vi "Display Error.vi"(8 "error in (no error)":errorcluster, 11 "Application Manager":refnum<k7>) -> (0 "error out":errorcluster)   [LabVIEW 2010, in "TS Simple LabVIEW OI Dependencies.lvlib"]
uses:
  TS Simple LabVIEW OI Dependencies.lvlib
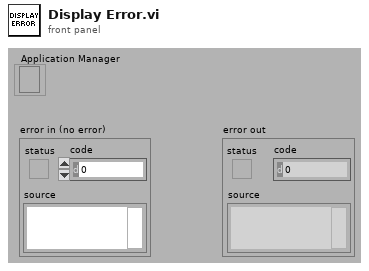
[diagram p1: front panel]
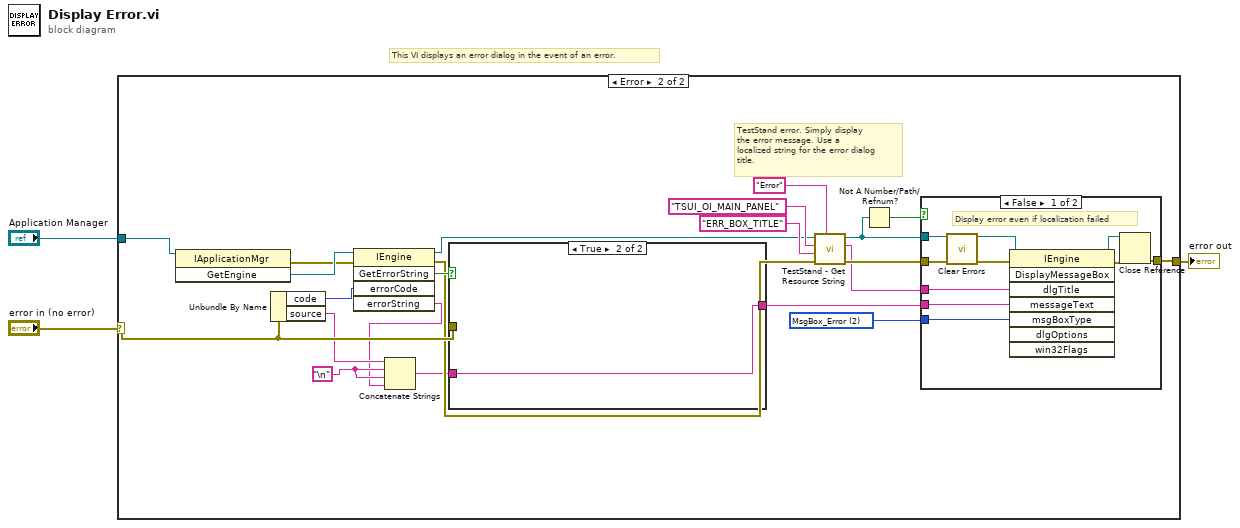
[diagram p0: block diagram]
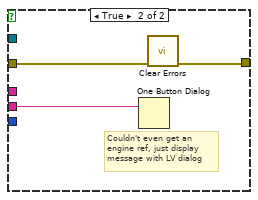
[diagram p3: hidden frame]
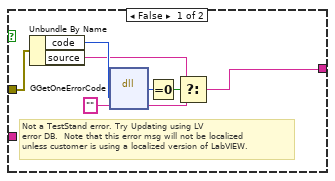
[diagram p4: hidden frame]
diagram:
  # "This VI displays an error dialog in the event of an error."
  n1 = case shown="Error" "error in (no error)" {
    selector: "error in (no error)" -> [w4 w24]
    tunnel: [w4 w16] -> w2
    tunnel: "Application Manager" -> [_ w17]
    frame No Error {
    }
    frame Error {
      w6 = "\n"
      w12 = 2 items=["MsgBox_Warning", "MsgBox_Information", "MsgBox_Error", "MsgBox_Custom"] ("msgBoxType")
      # "TestStand error. Simply display\nthe error message. Use a\nlocalized string for the error dialog\ntitle."
      n2 = invoke class="IApplicationMgr" method="GetEngine"(reference=w17) -> (error out=w22:errorcluster, "GetEngine"=w23:refnum<k7>)  [unwired: 2 in, 1 out]
      n3 = Unbundle By Name(w24) -> ("code"=w26:i32, "source"=w7:string)
      n4 = invoke class="IEngine" method="GetErrorString"(reference=w23, error in=w22, "errorCode"=w26) -> (reference out=w18:refnum<k7>, error out=w19:errorcluster, "GetErrorString"=w25:bool, "errorString"=w5:string)  [unwired: 2 in, 1 out]
      n5 = Concatenate Strings(w7, w6, w6, w5) -> (w8:string)
      n6 = case shown="True" w25 {
        tunnel: w24 -> [w40 _]
        tunnel: [w39 w47] -> w13
        tunnel: w8 -> [_ w47]
        frame False {
          # "Not a TestStand error. Try Updating using LV\nerror DB.  Note that this error msg will not be localized\nunless customer is using a localized version of LabVIEW."
          n7 = Unbundle By Name(w40) -> ("code"=w42:i32, "source"=w41:string)
          n8 = dll-call lib="LabVIEW" fn="GGetOneErrorCode"("errorCode"=w42, "" ("input param")) -> (w45:u8, w43:string)  [unwired: 4 in, 2 out]
          n9 = Equal To 0?(x=w45) -> (x = 0?=w44:bool)
          n10 = Select(t=w41, s=w44, f=w43) -> (s? t:f=w39:string)
        }
        frame True {
        }
      }
      n11 = call <vilib>:"TestStand - Get Resource String.vi"("Default String"="Error", "error in (no error)"=w19, "Symbol"="ERR_BOX_TITLE", "Category"="TSUI_OI_MAIN_PANEL", "Engine Reference In"=w18) -> ("error out"=w15:errorcluster, "Resource String"=w14:string, "Engine Reference Out"=w11:refnum<k7>)  [unwired: 4 out]
      n12 = Not A Number/Path/Refnum?(number/path/refnum=w11) -> (NaN/Path/Refnum?=w10:bool)
      n13 = case shown="False" w10 {
        tunnel: [w35 w36] -> w16
        tunnel: w12 -> [w34 _]
        tunnel: w14 -> [w33 _]
        tunnel: w11 -> [w32 _]
        tunnel: w15 -> [w28 w37]
        tunnel: w13 -> [w29 w38]
        frame False {
          # "Display error even if localization failed"
          n14 = call <vilib>:"Clear Errors.vi"("error in (no error)"=w28) -> ("error out"=w27:errorcluster)  [unwired: 6 out]
          n15 = invoke class="IEngine" method="DisplayMessageBox"(reference=w32, error in=w27, "dlgTitle"=w33, "messageText"=w29, "msgBoxType"=w34) -> (reference out=w30:refnum<k7>, error out=w31:errorcluster)  [unwired: 3 in, 6 out]
          n16 = Close Reference(reference=w30, error in (no error)=w31) -> (error out=w35:errorcluster)
        }
        frame True {
          # "Couldn't even get an\nengine ref, just display\nmessage with LV dialog"
          n17 = One Button Dialog(message=w38) -> ()  [unwired: 2 out]
          n18 = call <vilib>:"Clear Errors.vi"("error in (no error)"=w37) -> ("error out"=w36:errorcluster)  [unwired: 6 out]
        }
      }
    }
  }
  "error out" <- w2
